vi "DAQarm.vi"(8 "error in (no error)":errorcluster, 11 "DAQcamera in":refnum<class "DAQcamera.lvclass">) -> (0 "error out":errorcluster, 3 "DAQcamera out":refnum<class "DAQcamera.lvclass">)   [LabVIEW 2016, in "DAQcamera.lvclass"]
uses:
  DAQcamera.lvclass
  C:/Users/curtis.gutjahr/Documents/Labview Code/CTControl Code/PI Utilities/DAQclass/DAQdevice/DAQdevice.lvclass
  <vilib>/userdefined/High Color/IMAQdx.ctl
  DAQdevice/DAQdevice.lvclass/DAQdevice.ctl
  DAQcamera.lvclass/DAQcamera.ctl
  <vilib>/vision/driver/NI_Vision_Acquisition_Software.lvlib
  DAQdevice/DAQdevice.lvclass
panel:
  out "error out 2":errorcluster
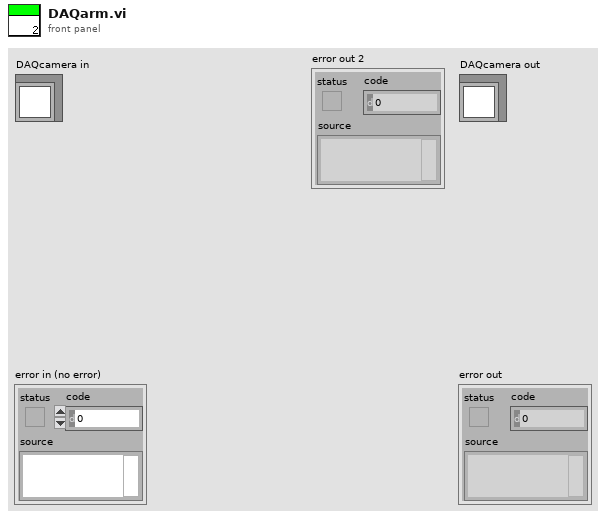
[diagram p1: front panel]
types:
  T1 = typedef "IMAQdx.ctl" = refnum<k21>
  T2 = cluster{"Type":u32, "Version":u32, "Flags":u32, "SerialNumberHigh":u32, "SerialNumberLow":u32, "BusType":u32, "InterfaceName":string, "VendorName":string, "ModelName":string, "CameraFileName":string, "CameraAttributeURL":string}
  T3 = cluster{"Type":u32, "Version":u32, "Flags":u32, "SerialNumberHigh":u32, "SerialNumberLow":u32, "BusType":u32, "InterfaceName":string, "VendorName":string, "ModelName":string, "CameraFileName":string, "CameraAttributeURL":string}[]
  T4 = typedef "IMAQ Image.ctl" = refnum<image>
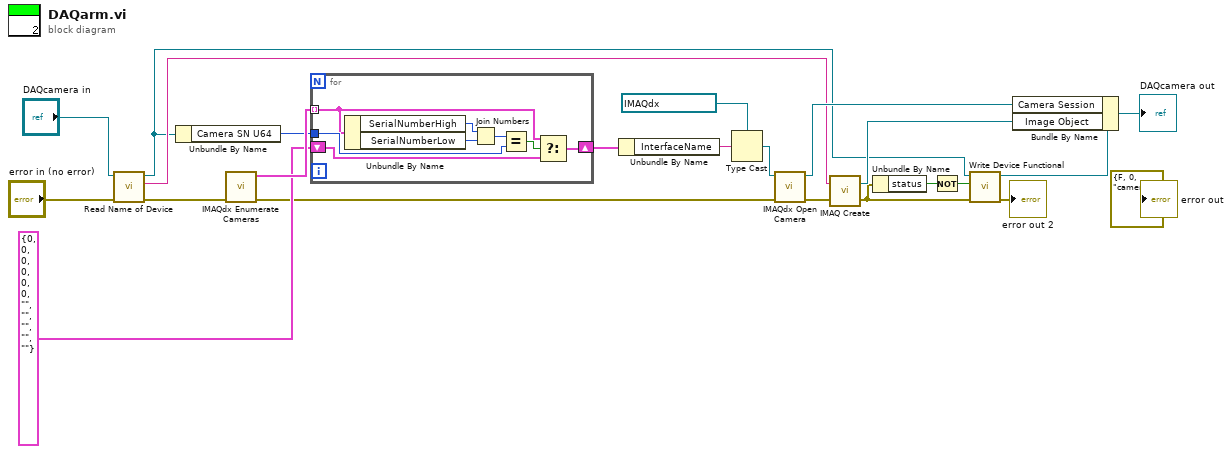
[diagram p0: block diagram]
diagram:
  n1 = call "Read Name of Device.vi"("error in (no error)"="error in (no error)", "DAQdevice in"="DAQcamera in") -> ("error out"=w4:errorcluster, "Name of Device"=w10:string, "DAQdevice out"=w9:refnum<class "DAQcamera.lvclass">)  [unwired: 7 in]
  n2 = Unbundle By Name(w9) -> ("Camera SN U64"=w14:u64)
  n3 = call <vilib>:"IMAQdx Enumerate Cameras.vi"("error in"=w4) -> ("error out"=w13:errorcluster, "Camera Information Array"=w23:T3)  [unwired: 9 in]
  n4 = for {
    tunnel: w23 -> [w24] mode=indexing
    tunnel: w14 -> [w28]
    shift-right: [w26] -> w21
    shift-left: T2 {"Type"=0, "Version"=0, "Flags"=0, "SerialNumberHigh"=0, "SerialNumberLow"=0, "BusType"=0, "InterfaceName"="", "VendorName"="", "ModelName"="", "CameraFileName"="", "CameraAttributeURL"=""} ("Cluster 3") -> [w25]
    n5 = Unbundle By Name(w24) -> ("SerialNumberHigh"=w31:u32, "SerialNumberLow"=w30:u32)
    n6 = Join Numbers(hi=w31, lo=w30) -> ((hi.lo)=w29:u64)
    n7 = Equal?(x=w29, y=w28) -> (x = y?=w27:bool)
    n8 = Select(t=w24, s=w27, f=w25) -> (s? t:f=w26:T2)
  }
  n9 = Unbundle By Name(w21) -> ("InterfaceName"=w12:string)
  n10 = Type Cast(type=T1 "CapVoltCam" ("Camera Name"), x=w12) -> (*(type *) &x=w19:T1)
  n11 = call <vilib>:"IMAQdx Open Camera.vi"("error in"=w13, "Session In"=w19) -> ("error out"=w17:errorcluster, "Session Out"=w18:T1)  [unwired: 8 in]
  n12 = call "IMAQ Create"("Image Name"=w10, "error in (no error)"=w17) -> ("New Image"=w16:T4, "error out"=w3:errorcluster)  [unwired: 2 in, 1 out]
  n13 = Unbundle By Name(w3) -> ("status"=w15:bool)
  n14 = Not(x=w15) -> (.not. x?=w8:bool)
  n15 = call "Write Device Functional.vi"("error in (no error)"=w3, "Device Functional"=w8, "DAQdevice in"=w9) -> ("error out"=→"error out 2":errorcluster, "DAQdevice out"=w7:refnum<class "DAQcamera.lvclass">)  [unwired: 7 in]
  n16 = Bundle By Name(cluster=w7, "Camera Session"=w18, "Image Object"=w16) -> (→"DAQcamera out":refnum<class "DAQcamera.lvclass">)
  "error out" <- errorcluster {"status"=FALSE, "code"=0, "source"="camera"} ("error out")
